vi "StepperLauncher.vi"   [LabVIEW 2014]
uses:
  Project/Implementations/Hardware/Real Hardware/ParameterDevice/Stepper3D/Stepper3D.lvclass
  <vilib>/ActorFramework/Actor/Actor.lvclass
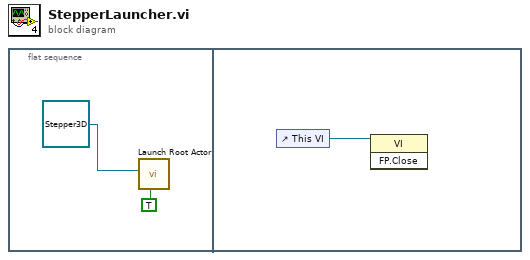
[diagram p0: block diagram]
diagram:
  n1 = flat-sequence {
    frame #0 {
      n2 = call <vilib>:"Launch Root Actor.vi"("Open Actor Core front panel? (F)"=TRUE, "Actor"=refnum<class "Stepper3D.lvclass"> refnum ("Stepper3D.lvclass")) -> ()  [unwired: 8 in, 2 out]
    }
    frame #1 {
      n3 = control-ref of="This VI"() -> (w3:refnum<vi>)
      n4 = invoke class="VI" method="FP.Close"(reference=w3) -> ()  [unwired: 2 in, 3 out]
    }
  }
